vi "BRig_RT_comm_tcp_write_RTwrite__RunState_Trial_selResult__v3.vi"(7 "input_dataTrial":u16[][](array[numeric]), 10 "iReward_or_iError":bool, 11 "input_dataCurrent":u16[](array[numeric])) -> (2 "output_strCmd":string)   [LabVIEW 2014]
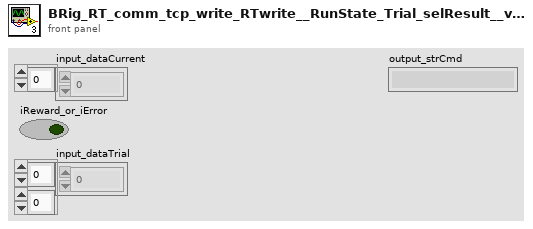
[diagram p1: front panel]
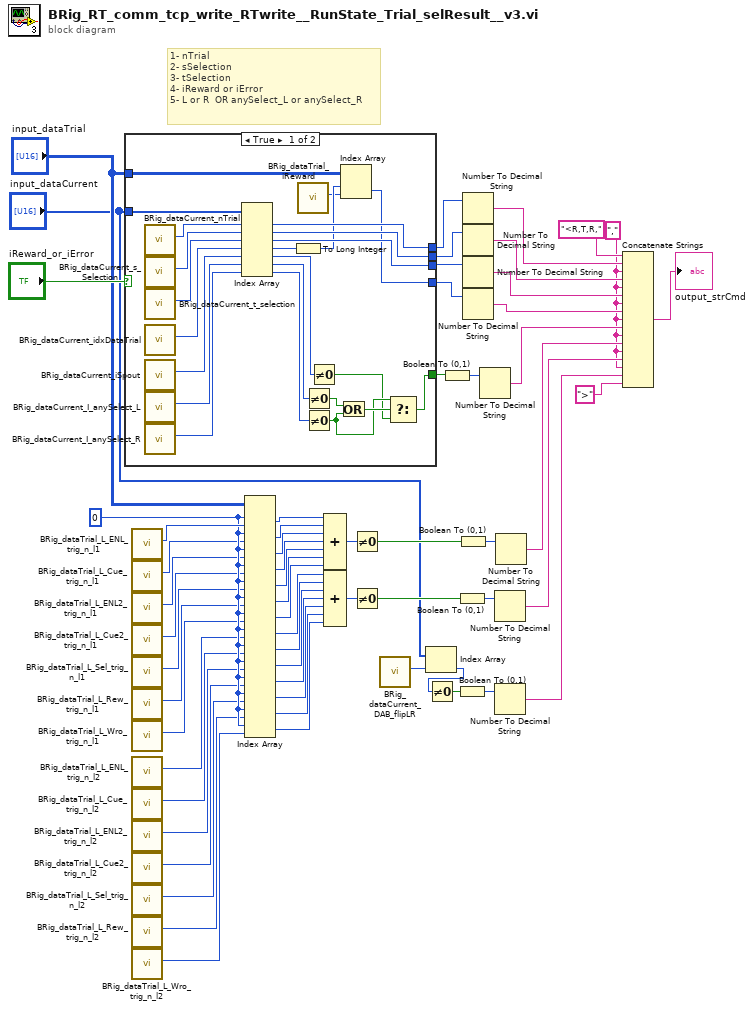
[diagram p0: block diagram]
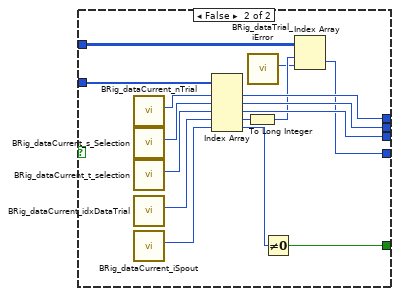
[diagram p2: hidden frame]
diagram:
  w36 = 0
  w7 = "," ("string")
  # "1- nTrial\n2- sSelection\n3- tSelection\n4- iReward or iError\n5- L or R  OR anySelect_L or anySelect_R"
  n1 = case shown="True" "iReward_or_iError" {
    tunnel: "input_dataCurrent" -> [w83 w99]
    tunnel: [w80 w96] -> w55
    tunnel: [w79 w95] -> w54
    tunnel: [w78 w94] -> w53
    tunnel: "input_dataTrial" -> [w74 w90]
    tunnel: [w72 w89] -> w52
    tunnel: [w61 w86] -> w57
    frame True {
      n2 = call "BRig_dataCurrent_nTrial.vi"() -> ("output_nTrial"=w84:i32)  [unwired: 11 in]
      n3 = call "BRig_dataCurrent_s_Selection.vi"() -> ("output_s_Selection"=w82:i32)  [unwired: 11 in]
      n4 = call "BRig_dataCurrent_t_selection.vi"() -> ("output_t_selection"=w81:i32)  [unwired: 11 in]
      n5 = call "BRig_dataCurrent_idxDataTrial.vi"() -> ("output_idxDataTrial"=w77:i32)  [unwired: 11 in]
      n6 = call "BRig_dataCurrent_iSpout.vi"() -> ("output_iSpout"=w71:i32)  [unwired: 11 in]
      n7 = call "BRig_dataCurrent_I_anySelect_L.vi"() -> ("output_IanySelect_L"=w70:i32)  [unwired: 11 in]
      n8 = call "BRig_dataCurrent_I_anySelect_R.vi"() -> ("output_IanySelect_R"=w69:i32)  [unwired: 11 in]
      n9 = Index Array(array=w83, index #1=w84, index #2=w82, index #3=w81, index #4=w77, index #5=w71, index #6=w70, index #7=w69) -> (element #1=w80:u16, element #2=w79:u16, element #3=w78:u16, element #4=w76:u16, element #5=w63:u16, element #6=w68:u16, element #7=w67:u16)
      n10 = To Long Integer(number=w76) -> (32bit integer=w75:i32)
      n11 = call "BRig_dataTrial_iReward.vi"() -> ("output_iReward"=w73:i32)  [unwired: 11 in]
      n12 = Not Equal To 0?(x=w68) -> (x != 0?=w66:bool)
      n13 = Not Equal To 0?(x=w67) -> (x != 0?=w64:bool)
      n14 = Not Equal To 0?(x=w63) -> (x != 0?=w62:bool)
      n15 = Or(x=w66, y=w64) -> (x .or. y?=w65:bool)
      n16 = Index Array(array=w74, index (row)=w75, index (col)=w73) -> (element=w72:u16)
      n17 = Select(t=w64, s=w65, f=w62) -> (s? t:f=w61:bool)
    }
    frame False {
      n18 = call "BRig_dataCurrent_nTrial.vi"() -> ("output_nTrial"=w100:i32)  [unwired: 11 in]
      n19 = call "BRig_dataCurrent_s_Selection.vi"() -> ("output_s_Selection"=w98:i32)  [unwired: 11 in]
      n20 = call "BRig_dataCurrent_t_selection.vi"() -> ("output_t_selection"=w97:i32)  [unwired: 11 in]
      n21 = call "BRig_dataCurrent_idxDataTrial.vi"() -> ("output_idxDataTrial"=w93:i32)  [unwired: 11 in]
      n22 = call "BRig_dataCurrent_iSpout.vi"() -> ("output_iSpout"=w88:i32)  [unwired: 11 in]
      n23 = Index Array(array=w99, index #1=w100, index #2=w98, index #3=w97, index #4=w93, index #5=w88) -> (element #1=w96:u16, element #2=w95:u16, element #3=w94:u16, element #4=w92:u16, element #5=w87:u16)
      n24 = To Long Integer(number=w92) -> (32bit integer=w91:i32)
      n25 = call "BRig_dataTrial_iError.vi"() -> ("output_iError"=w85:i32)  [unwired: 11 in]
      n26 = Not Equal To 0?(x=w87) -> (x != 0?=w86:bool)
      n27 = Index Array(array=w90, index (row)=w91, index (col)=w85) -> (element=w89:u16)
    }
  }
  n28 = call "BRig_dataTrial_L_ENL_trig_n_l1.vi"() -> ("output_L_ENL_trig_n_l1"=w37:i32)  [unwired: 11 in]
  n29 = call "BRig_dataTrial_L_Cue_trig_n_l1.vi"() -> ("output_L_Cue_trig_n_l1"=w35:i32)  [unwired: 11 in]
  n30 = call "BRig_dataTrial_L_ENL2_trig_n_l1.vi"() -> ("output_L_ENL2_trig_n_l1"=w34:i32)  [unwired: 11 in]
  n31 = call "BRig_dataTrial_L_Cue2_trig_n_l1.vi"() -> ("output_L_Cue2_trig_n_l1"=w33:i32)  [unwired: 11 in]
  n32 = call "BRig_dataTrial_L_Sel_trig_n_l1.vi"() -> ("output_L_Sel_trig_n_l1"=w32:i32)  [unwired: 11 in]
  n33 = call "BRig_dataTrial_L_Rew_trig_n_l1.vi"() -> ("output_L_Reward_trig_n_l1"=w12:i32)  [unwired: 11 in]
  n34 = call "BRig_dataTrial_L_Wro_trig_n_l1.vi"() -> ("output_L_Wrong_trig_n_l1"=w10:i32)  [unwired: 11 in]
  n35 = call "BRig_dataTrial_L_ENL_trig_n_l2.vi"() -> ("output_L_ENL_trig_n_l2"=w31:i32)  [unwired: 11 in]
  n36 = call "BRig_dataTrial_L_Cue_trig_n_l2.vi"() -> ("output_L_Cue_trig_n_l2"=w30:i32)  [unwired: 11 in]
  n37 = call "BRig_dataTrial_L_ENL2_trig_n_l2.vi"() -> ("output_L_ENL2_trig_n_l2"=w29:i32)  [unwired: 11 in]
  n38 = call "BRig_dataTrial_L_Cue2_trig_n_l2.vi"() -> ("output_L_Cue2_trig_n_l2"=w28:i32)  [unwired: 11 in]
  n39 = call "BRig_dataTrial_L_Sel_trig_n_l2.vi"() -> ("output_L_Sel_trig_n_l2"=w27:i32)  [unwired: 11 in]
  n40 = call "BRig_dataTrial_L_Rew_trig_n_l2.vi"() -> ("output_L_Reward_trig_n_l2"=w11:i32)  [unwired: 11 in]
  n41 = call "BRig_dataTrial_L_Wro_trig_n_l2.vi"() -> ("output_L_Wrong_trig_n_l2"=w9:i32)  [unwired: 11 in]
  n42 = Index Array(array="input_dataTrial", index (row) #1=w36, index (col) #1=w37, index (row) #2=w36, index (col) #2=w35, index (row) #3=w36, index (col) #3=w34, index (row) #4=w36, index (col) #4=w33, index (row) #5=w36, index (col) #5=w32, index (row) #6=w36, index (col) #6=w12, index (row) #7=w36, index (col) #7=w10, index (row) #8=w36, index (col) #8=w31, index (row) #9=w36, index (col) #9=w30, index (row) #10=w36, index (col) #10=w29, index (row) #11=w36, index (col) #11=w28, index (row) #12=w36, index (col) #12=w27, index (row) #13=w36, index (col) #13=w11, index (row) #14=w36, index (col) #14=w9) -> (element #1=w26:u16, element #2=w25:u16, element #3=w24:u16, element #4=w23:u16, element #5=w22:u16, element #6=w21:u16, element #7=w20:u16, element #8=w19:u16, element #9=w18:u16, element #10=w17:u16, element #11=w16:u16, element #12=w15:u16, element #13=w14:u16, element #14=w13:u16)
  n43 = Compound Arithmetic op=ADD(w26, w25, w24, w23, w22, w21, w20) -> (w46:u16)
  n44 = Compound Arithmetic op=ADD(w19, w18, w17, w16, w15, w14, w13) -> (w45:u16)
  n45 = Not Equal To 0?(x=w46) -> (x != 0?=w42:bool)
  n46 = Not Equal To 0?(x=w45) -> (x != 0?=w41:bool)
  n47 = call "BRig_dataCurrent_DAB_flipLR.vi"() -> ("output_DAB_flipLR"=w1:i32)  [unwired: 11 in]
  n48 = Index Array(array="input_dataCurrent", index=w1) -> (element=w3:u16)
  n49 = Not Equal To 0?(x=w3) -> (x != 0?=w6:bool)
  n50 = Boolean To (0,1)(Boolean=w57) -> (0, 1=w56:i16)
  n51 = Boolean To (0,1)(Boolean=w41) -> (0, 1=w43:i16)
  n52 = Boolean To (0,1)(Boolean=w6) -> (0, 1=w5:i16)
  n53 = Boolean To (0,1)(Boolean=w42) -> (0, 1=w44:i16)
  n54 = Number To Decimal String(number=w55) -> (decimal integer string=w51:string)  [unwired: 1 in]
  n55 = Number To Decimal String(number=w54) -> (decimal integer string=w50:string)  [unwired: 1 in]
  n56 = Number To Decimal String(number=w53) -> (decimal integer string=w49:string)  [unwired: 1 in]
  n57 = Number To Decimal String(number=w52) -> (decimal integer string=w48:string)  [unwired: 1 in]
  n58 = Number To Decimal String(number=w56) -> (decimal integer string=w47:string)  [unwired: 1 in]
  n59 = Number To Decimal String(number=w43) -> (decimal integer string=w39:string)  [unwired: 1 in]
  n60 = Number To Decimal String(number=w5) -> (decimal integer string=w2:string)  [unwired: 1 in]
  n61 = Number To Decimal String(number=w44) -> (decimal integer string=w40:string)  [unwired: 1 in]
  n62 = Concatenate Strings("<R,T,R," ("string"), w51, w7, w50, w7, w49, w7, w48, w7, w47, w7, w40, w7, w39, w7, w2, ">" ("string")) -> (→"output_strCmd":string)
